vi "pp3b_DAQinit.vi"(8 "error in (no error)":errorcluster, 11 "Daq config in":T1={"Sound AO"="Dev6/ao0", "Shock intesity AO"="Dev6/ao1", "Code_LED DO"="Dev6/port1:2", "Switch DI"="Dev6/port0/line0", "Webcam"="cam9", "Sound AO task"="", "Sound card task"=0, "Shock intensity AO task"="", "Code_LED DO task"="", "Switch DI task"="", "AO <=> Sound card"=FALSE, "Sound card"=0, "sample rate"=100000.0, "Variable shock"=TRUE, "Webcam on"=FALSE, "Waveform memo"={"t0"=timestamp(0 s since 1904-01-01), "dt"=1.0, "Y"=[]}, "First time"=FALSE, "Tone trigger"="PFI1", "Master-9 DO"="Dev6/port0/line5:7", "Master-9 DO task"=""} {"sample rate" min=8000.0; "Sound card task" format="%.0x"}) -> (0 "error out":errorcluster={"status"=FALSE, "code"=0, "source"="\n"}, 3 "Daq config out":T1={"Sound AO"="Dev6/ao0", "Shock intesity AO"="Dev6/ao1", "Code_LED DO"="Dev6/port1:2", "Switch DI"="Dev6/port0/line0", "Webcam"="cam9", "Sound AO task"="", "Sound card task"=0, "Shock intensity AO task"="", "Code_LED DO task"="", "Switch DI task"="", "AO <=> Sound card"=FALSE, "Sound card"=0, "sample rate"=100000.0, "Variable shock"=TRUE, "Webcam on"=FALSE, "Waveform memo"={"t0"=timestamp(0 s since 1904-01-01), "dt"=1.0, "Y"=[]}, "First time"=FALSE, "Tone trigger"="PFI1", "Master-9 DO"="Dev6/port0/line5:7", "Master-9 DO task"=""} {"sample rate" min=8000.0; "Sound card task" format="%.0x"})   [LabVIEW 2013]
uses:
  <vilib>/DAQmx/create/channels.llb/DAQmx Create Channel (AO-Voltage-Basic).vi
  <vilib>/DAQmx/create/channels.llb/DAQmx Create Channel (DO-Digital Output).vi
  <vilib>/sound2/lvsound2.llb/Sampling Mode.ctl
  <vilib>/sound2/lvsound2.llb/Sound Output Task ID.ctl
  <vilib>/DAQmx/configure/timing.llb/DAQmx Timing (Sample Clock).vi
  <vilib>/sound2/lvsound2.llb/Sound Data Format.ctl
  <vilib>/DAQmx/create/channels.llb/DAQmx Create Channel (DI-Digital Input).vi
  <resource>/objmgr/daqmx.rc
  <vilib>/DAQmx/write.llb/DAQmx Write (Digital U16 1Chan 1Samp).vi
  <vilib>/DAQmx/write.llb/DAQmx Write (Digital U32 1Chan 1Samp).vi
  <vilib>/userdefined/High Color/IMAQdx.ctl
  pp3c_CTL_DaqStatusVariable.ctl
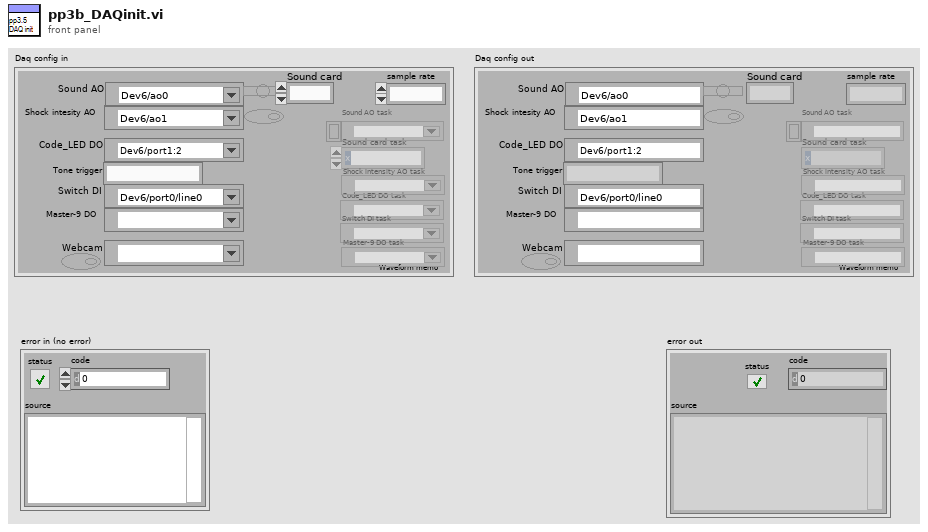
[diagram p1: front panel]
types:
  T1 = typedef "pp3c_CTL_DaqStatusVariable.ctl" = cluster{"Sound AO":tag, "Shock intesity AO":tag, "Code_LED DO":tag, "Switch DI":tag, "Webcam":T2, "Sound AO task":refnum<k21>, "Sound card task":T3, "Shock intensity AO task":refnum<k21>, "Code_LED DO task":refnum<k21>, "Switch DI task":refnum<k21>, "AO <=> Sound card":bool, "Sound card":u32, "sample rate":dbl, "Variable shock":bool, "Webcam on":bool, "Waveform memo":waveform(dbl), "First time":bool, "Tone trigger":string, "Master-9 DO":tag, "Master-9 DO task":refnum<k21>}
  T2 = typedef "IMAQdx.ctl" = refnum<k21>
  T3 = typedef "Sound Output Task ID.ctl" = u32
  T4 = typedef "Sound Data Format.ctl" = cluster{"sample rate (S/s)":dbl, "number of channels":i32, "bits per sample":i32}
  T5 = typedef "Sampling Mode.ctl" = i32
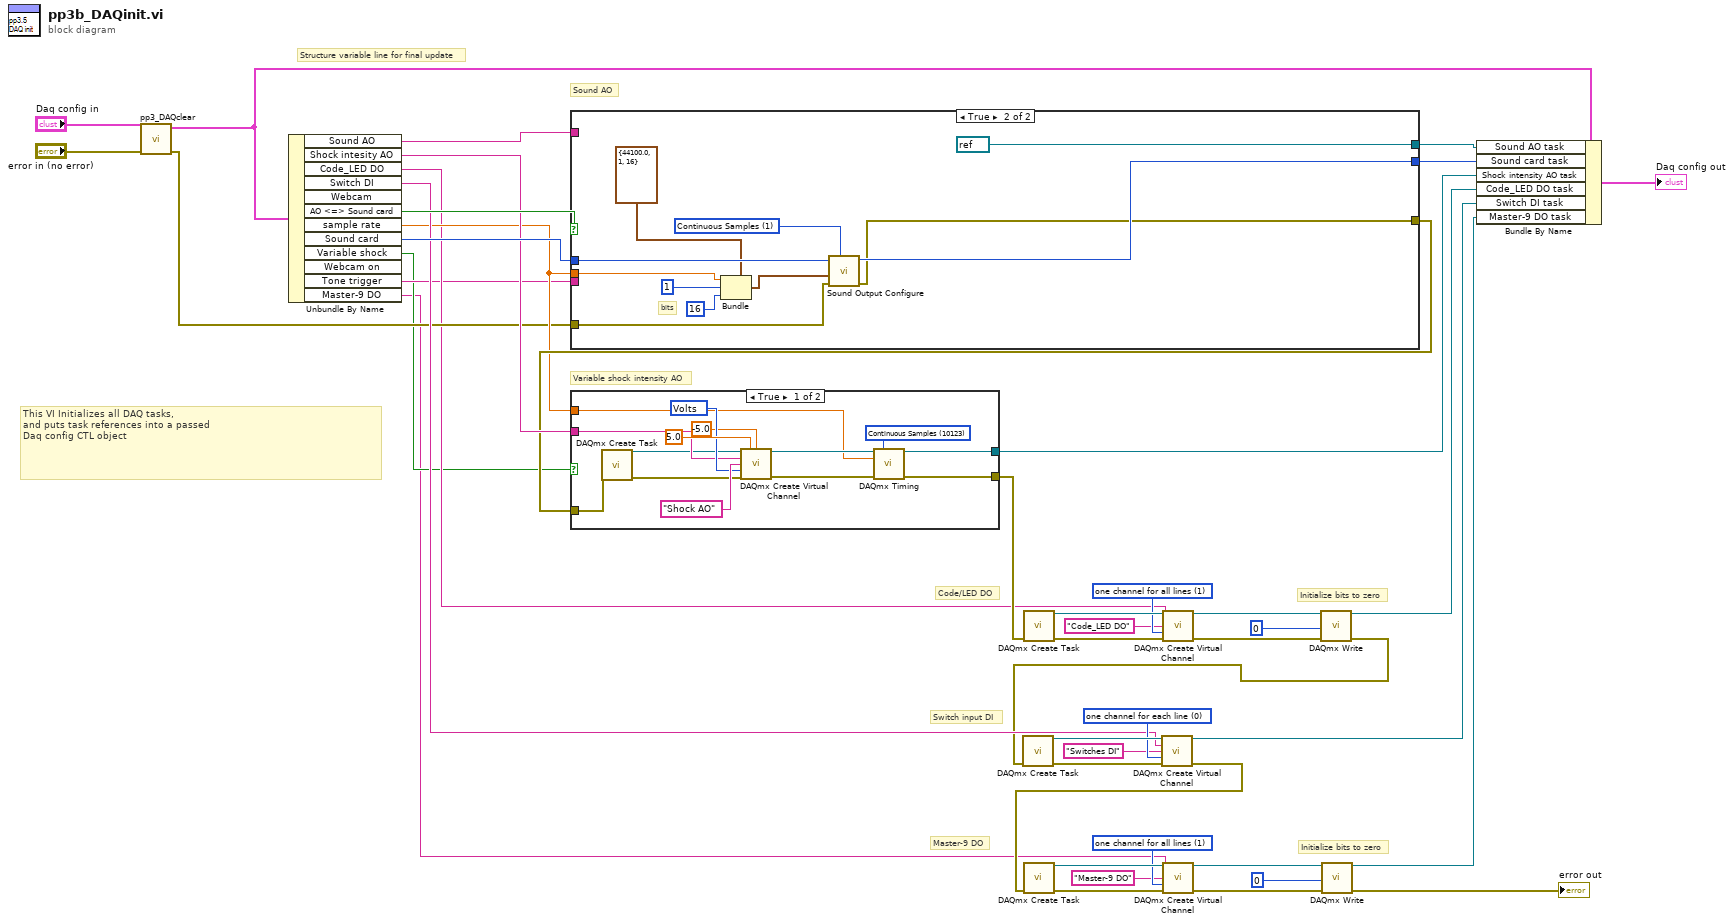
[diagram p0: block diagram]
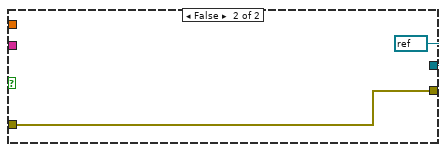
[diagram p2: hidden frame]
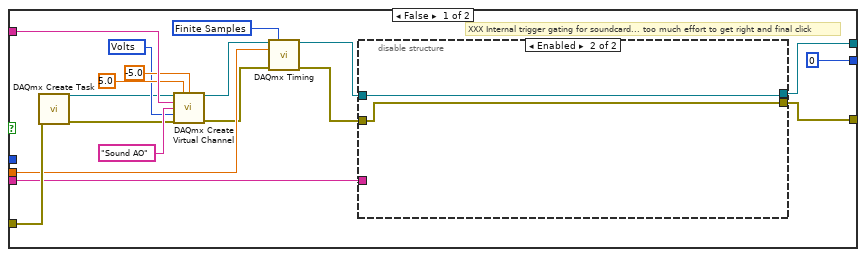
[diagram p3: hidden frame]
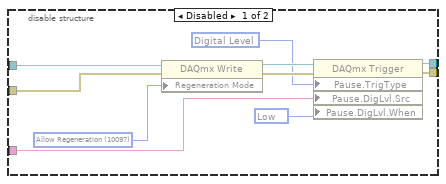
[diagram p4: hidden frame]
diagram:
  w14 = 1 items=["one channel for each line", "one channel for all lines"] ("line grouping")
  w30 = 0 items=["one channel for each line", "one channel for all lines"] ("line grouping")
  w34 = 1 items=["one channel for each line", "one channel for all lines"] ("line grouping")
  # "Initialize bits to zero"
  # "Initialize bits to zero"
  # "This VI Initializes all DAQ tasks,\nand puts task references into a passed\nDaq config CTL object"
  # "Switch input DI"
  # "Master-9 DO"
  # "Structure variable line for final update"
  # "Code/LED DO"
  # "Variable shock intensity AO"
  # "Sound AO"
  n1 = call "pp3_DAQclear.vi"("error in (no error)"="error in (no error)", "Daq config in"="Daq config in") -> ("error out"=w20:errorcluster, "Daq config out"=w22:T1)  [unwired: 8 in]
  n2 = Unbundle By Name(w22) -> ("Sound AO"=w43:tag, "Shock intesity AO"=w38:tag, "Code_LED DO"=w19:tag, "Switch DI"=w28:tag, "AO <=> Sound card"=w44:bool, "sample rate"=w24:dbl, "Sound card"=w40:u32, "Variable shock"=w17:bool, "Tone trigger"=w18:string, "Master-9 DO"=w11:tag)  [unwired: 2 out]
  n3 = case shown="True" w44 {
    tunnel: w43 -> [w62 _]
    tunnel: [w52 refnum<k21> refnum ("task out")] -> w41
    tunnel: w40 -> [_ w84]
    tunnel: [T3 0 ("task ID") w80] -> w39
    tunnel: w20 -> [w56 w79]
    tunnel: [w51 w78] -> w26
    tunnel: w24 -> [w49 w77]
    tunnel: w18 -> [w53 _]
    frame False {
      w46 = 10178 items=["Finite Samples"=10178, "Continuous Samples"=10123, "Hardware Timed Single Point"=12522] ("sample mode")
      w57 = 10348 items=["Volts"=10348, "From Custom Scale"=10065] ("units")
      # "XXX Internal trigger gating for soundcard... too much effort to get right and final click"
      n4 = call <vilib>:"DAQmx Create Task.vi"("error in"=w56) -> ("task out"=w55:refnum<k21>, "error out"=w54:errorcluster)  [unwired: 13 in]
      n5 = call-poly <vilib>:"DAQmx Create Virtual Channel.vi"("task in"=w55, "maximum value"=5.0, "minimum value"=-5.0, "physical channels"=w62, "name to assign"="Sound AO", "units"=w57, "error in"=w54) -> ("task out"=w50:refnum<k21>, "error out"=w48:errorcluster)  [unwired: 7 in]
      n6 = call-poly <vilib>:"DAQmx Timing.vi"("task/channels in"=w50, "sample mode"=w46, "rate"=w49, "error in"=w48) -> ("task out"=w45:refnum<k21>, "error out"=w47:errorcluster)  [unwired: 10 in]
      n7 = disable-structure shown="Enabled" {
        disable-tunnel: w45 -> [w71 w74]
        disable-tunnel: w47 -> [w70 w73]
        disable-tunnel: w53 -> [w66 _]
        disable-tunnel: [w64 w74] -> w52
        disable-tunnel: [w63 w73] -> w51
        frame Disabled {
          w69 = 10214 items=["High"=10192, "Low"=10214] ("Pause.DigLvl.When")
          w65 = 10152 items=["Analog Level"=10101, "Analog Window"=10103, "Digital Level"=10152, "Digital Pattern"=10398, "None"=10230] ("Pause.TrigType")
          w72 = 10097 items=["Allow Regeneration"=10097, "Do Not Allow Regeneration"=10158] ("RegenMode")
          n8 = property class="DAQmx Write"(reference=w71, error in=w70, "Regeneration Mode"=w72) -> (reference out=w68:refnum<k21>, error out=w67:errorcluster)
          n9 = property class="DAQmx Trigger"(reference=w68, error in=w67, "Pause.TrigType"=w65, "Pause.DigLvl.Src"=w66, "Pause.DigLvl.When"=w69) -> (reference out=w64:refnum<k21>, error out=w63:errorcluster)
        }
        frame Enabled {
        }
      }
    }
    frame True {
      w83 = T5 1 items=["Finite Samples", "Continuous Samples"] ("sample mode")
      # "bits"
      n10 = Bundle(cluster=T4 {"sample rate (S/s)"=44100.0, "number of channels"=1, "bits per sample"=16} ("sound format"), "sample rate (S/s)"=w77, "number of channels"=1 ("Input.BufSize"), "bits per sample"=16 ("Input.BufSize")) -> (w75:T4)
      n11 = call <vilib>:"Sound Output Configure.vi"("sample mode"=w83, "error in (no error)"=w79, "sound format"=w75, "device ID"=w84) -> ("error out"=w78:errorcluster, "task ID"=w80:T3)  [unwired: 6 in]
    }
  }
  n12 = case shown="True" w17 {
    tunnel: w38 -> [w96 _]
    tunnel: [w90 refnum<k21> refnum ("task out")] -> w37
    tunnel: w24 -> [w92 _]
    tunnel: w26 -> [w88 w101]
    tunnel: [w89 w101] -> w25
    frame True {
      w91 = 10123 items=["Finite Samples"=10178, "Continuous Samples"=10123, "Hardware Timed Single Point"=12522] ("sample mode")
      w97 = 10348 items=["Volts"=10348, "From Custom Scale"=10065] ("units")
      n13 = call <vilib>:"DAQmx Create Task.vi"("error in"=w88) -> ("task out"=w86:refnum<k21>, "error out"=w87:errorcluster)  [unwired: 13 in]
      n14 = call-poly <vilib>:"DAQmx Create Virtual Channel.vi"("task in"=w86, "maximum value"=5.0, "minimum value"=-5.0, "physical channels"=w96, "name to assign"="Shock AO", "units"=w97, "error in"=w87) -> ("task out"=w94:refnum<k21>, "error out"=w93:errorcluster)  [unwired: 7 in]
      n15 = call-poly <vilib>:"DAQmx Timing.vi"("task/channels in"=w94, "sample mode"=w91, "rate"=w92, "error in"=w93) -> ("task out"=w90:refnum<k21>, "error out"=w89:errorcluster)  [unwired: 10 in]
    }
    frame False {
    }
  }
  n16 = call <vilib>:"DAQmx Create Task.vi"("error in"=w25) -> ("task out"=w35:refnum<k21>, "error out"=w36:errorcluster)  [unwired: 13 in]
  n17 = call-poly <vilib>:"DAQmx Create Virtual Channel.vi"("task in"=w35, "lines"=w19, "name to assign"="Code_LED DO", "line grouping"=w34, "error in"=w36) -> ("task out"=w10:refnum<k21>, "error out"=w8:errorcluster)  [unwired: 9 in]
  n18 = call-poly <vilib>:"DAQmx Write.vi"("task/channels in"=w10, "data"=u16 0, "error in"=w8) -> ("task out"=w9:refnum<k21>, "error out"=w6:errorcluster)  [unwired: 10 in, 1 out]
  n19 = call <vilib>:"DAQmx Create Task.vi"("error in"=w6) -> ("task out"=w31:refnum<k21>, "error out"=w32:errorcluster)  [unwired: 13 in]
  n20 = call-poly <vilib>:"DAQmx Create Virtual Channel.vi"("task in"=w31, "lines"=w28, "name to assign"="Switches DI", "line grouping"=w30, "error in"=w32) -> ("task out"=w27:refnum<k21>, "error out"=w12:errorcluster)  [unwired: 9 in]
  n21 = call <vilib>:"DAQmx Create Task.vi"("error in"=w12) -> ("task out"=w15:refnum<k21>, "error out"=w16:errorcluster)  [unwired: 13 in]
  n22 = call-poly <vilib>:"DAQmx Create Virtual Channel.vi"("task in"=w15, "lines"=w11, "name to assign"="Master-9 DO", "line grouping"=w14, "error in"=w16) -> ("task out"=w2:refnum<k21>, "error out"=w1:errorcluster)  [unwired: 9 in]
  n23 = call-poly <vilib>:"DAQmx Write.vi"("task/channels in"=w2, "data"=u32 0, "error in"=w1) -> ("task out"=w3:refnum<k21>, "error out"=→"error out":errorcluster)  [unwired: 10 in, 1 out]
  n24 = Bundle By Name(cluster=w22, "Sound AO task"=w41, "Sound card task"=w39, "Shock intensity AO task"=w37, "Code_LED DO task"=w9, "Switch DI task"=w27, "Master-9 DO task"=w3) -> (→"Daq config out":T1)
